vi "main.vi"() -> ()   [LabVIEW 2016]
uses:
  Typedefs/FGV_params.ctl
  Typedefs/FGV2_params.ctl
  Typedefs/State.ctl
  Typedefs/Acqstate.ctl
  <vilib>/Analysis/3filter.llb/Filter Passband Type.ctl
  <vilib>/DAQmx/read.llb/DAQmx Read (Analog 1D Wfm NChan NSamp).vi
  <vilib>/DAQmx/create/channels.llb/DAQmx Create Channel (AI-Voltage-Basic).vi
  <vilib>/DAQmx/configure/timing.llb/DAQmx Timing (Sample Clock).vi
  <vilib>/DAQmx/miscellaneous.llb/DAQmx Fill In Error Info.vi
  <vilib>/Analysis/3filter.llb/Butterworth Filter (DBL).vi
  <vilib>/Analysis/NI_AALBase.lvlib
panel:
  out "XZ":dbl(knob) scale=-90.0..90.0
  out "YZ":dbl(knob) scale=-90.0..90.0
  in  "Load?":bool
  in  "Save?":bool
  in  "Path?":path
  out "Acceleragement":waveform(dbl)[](graph)
  out "MAXY":dbl[](array[numeric])
  out "MINY":dbl[](array[numeric])
  in  "Axis?":string(combo)
  in  "Calibrate?":bool
  out "Voltagement":waveform(dbl)[](graph)
  in  "rate":dbl=1000.0 format="%0.2f"
  in  "samples per channel":i32=1000
  in  "stop":bool
  in  "Play?":bool
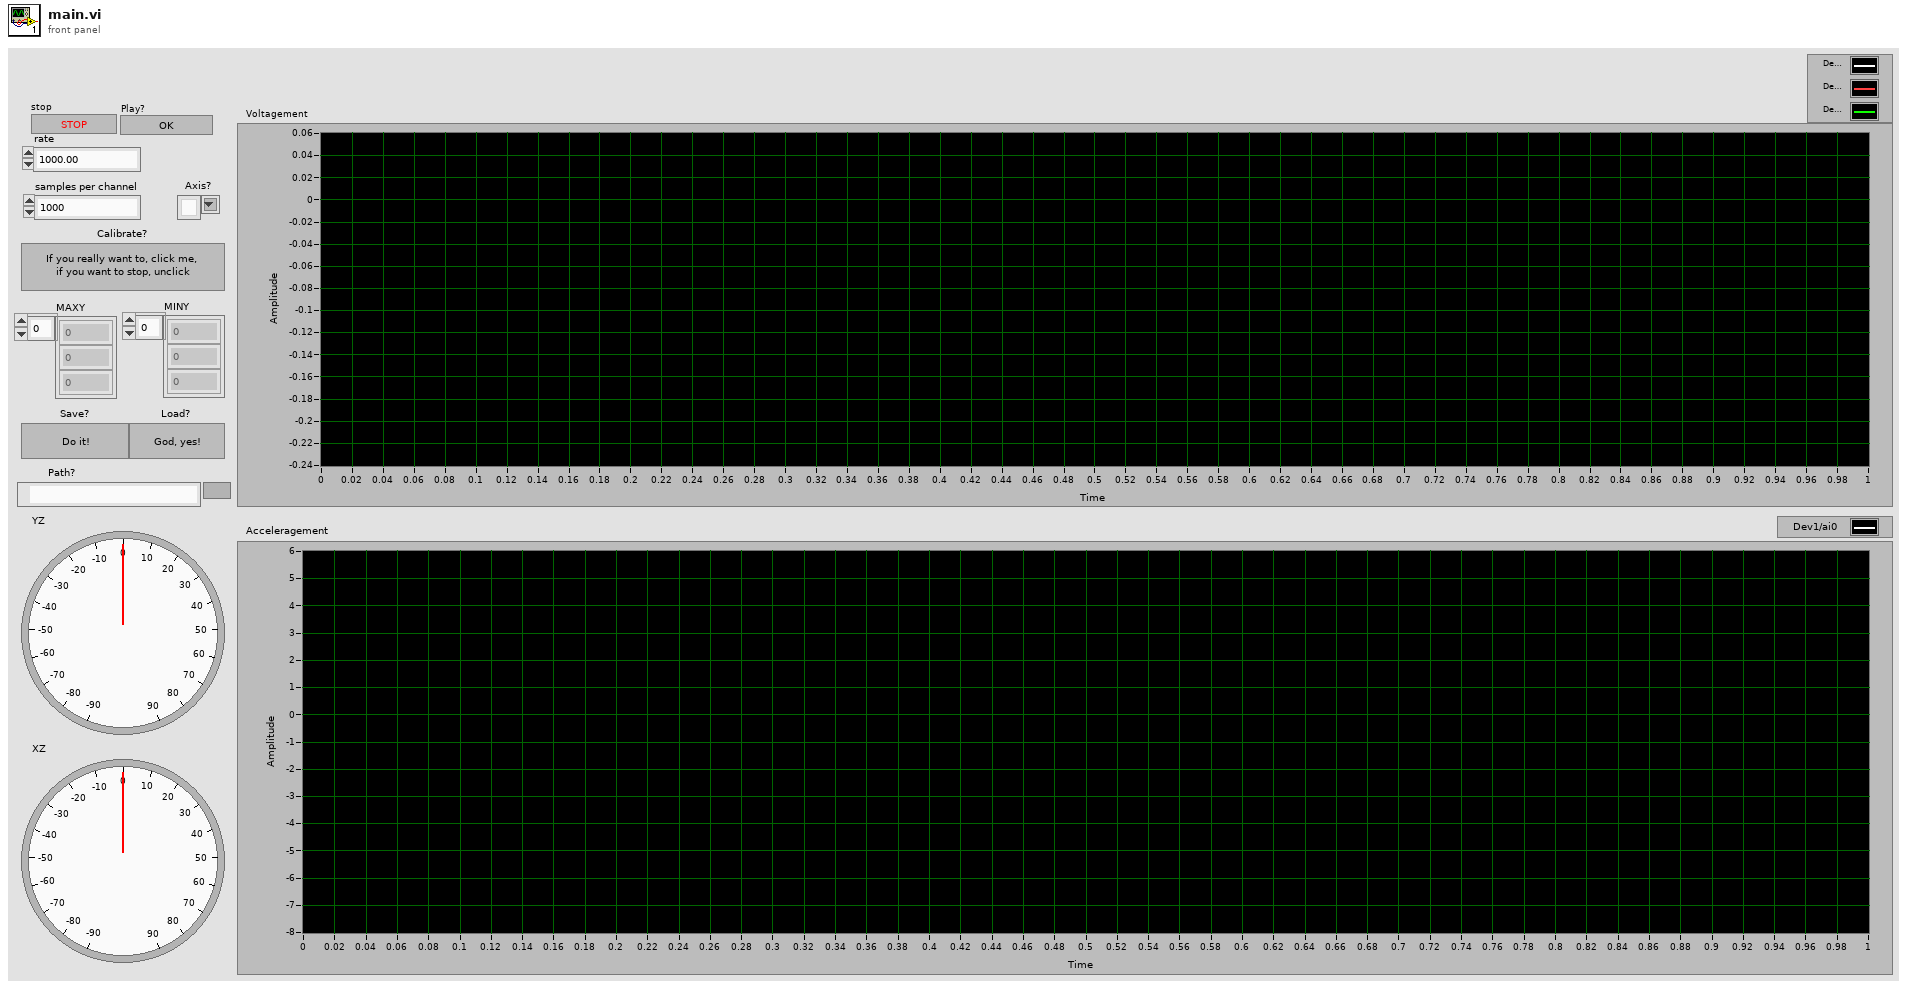
[diagram p1: front panel]
types:
  T1 = typedef "FGV2_params.ctl" = cluster{"Axis?":string, "Calibrate?":bool}
  T2 = typedef "FGV_params.ctl" = cluster{"Play":bool, "rate":dbl, "samples per channel":i32}
  T3 = typedef "Acqstate.ctl" = enum16{"Load", "Save", "Init", "Measurment", "Calibration"}
  T4 = typedef "State.ctl" = enum16{"Idel", "Init", "Acc", "End", ""}
  T5 = enum16{"open", "replace", "create", "open or create", "replace or create", "replace or create with confirmation"}
  T6 = typedef "NI_AALBase.lvlib/Filter Passband Type.ctl" = enum32{"Lowpass", "Highpass", "Bandpass", "Bandstop"}
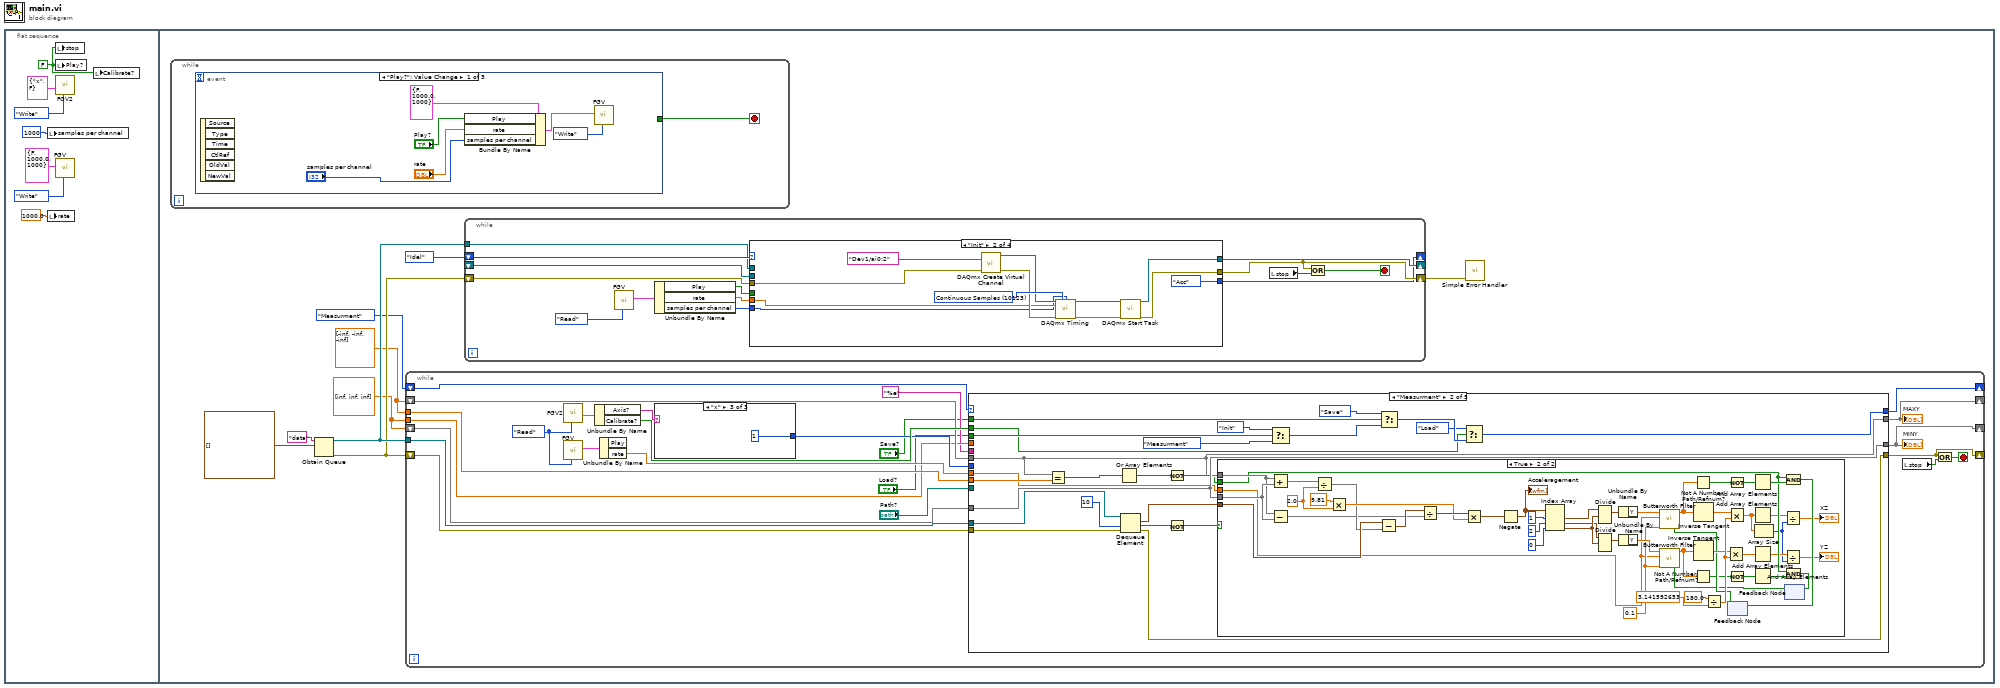
[diagram p0: block diagram]
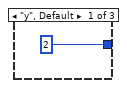
[diagram p2: hidden frame]
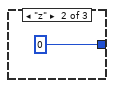
[diagram p3: hidden frame]
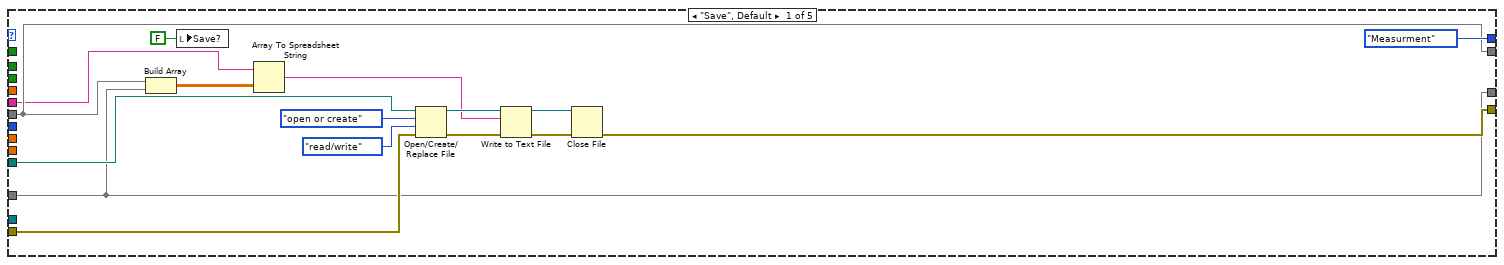
[diagram p4: hidden frame]
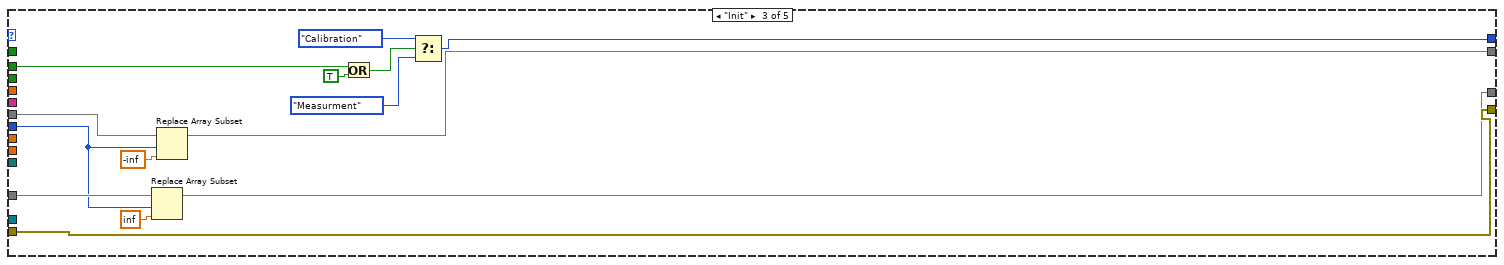
[diagram p6: hidden frame]
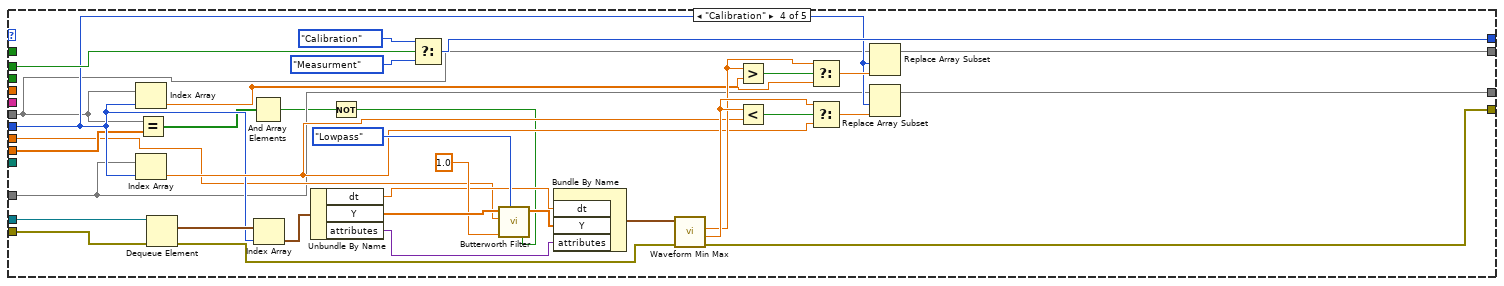
[diagram p7: hidden frame]
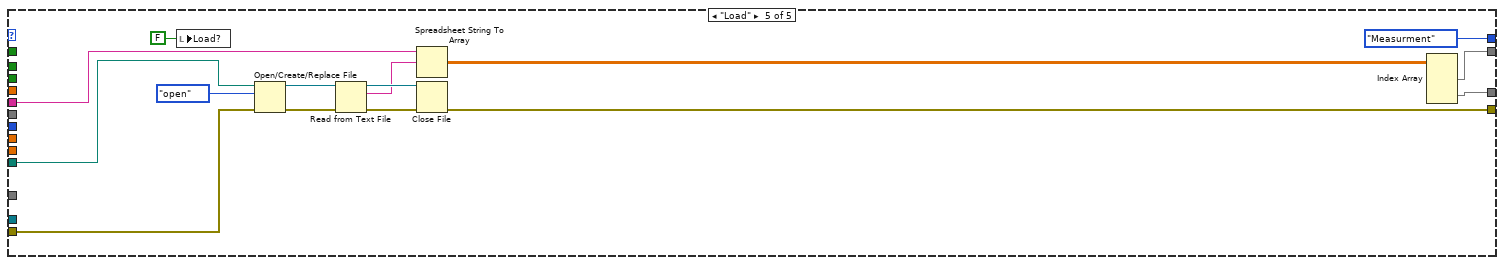
[diagram p8: hidden frame]
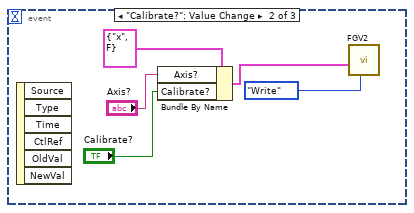
[diagram p9: hidden frame]
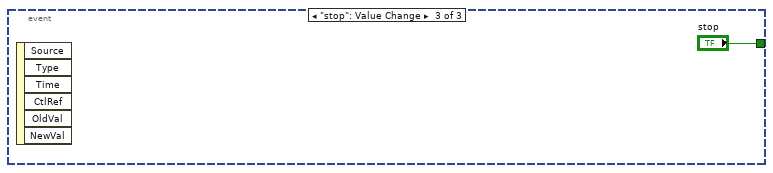
[diagram p10: hidden frame]
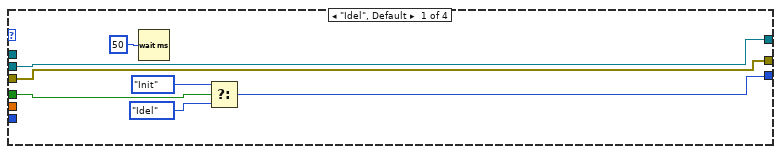
[diagram p11: hidden frame]
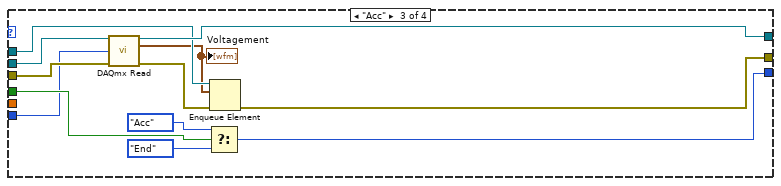
[diagram p12: hidden frame]
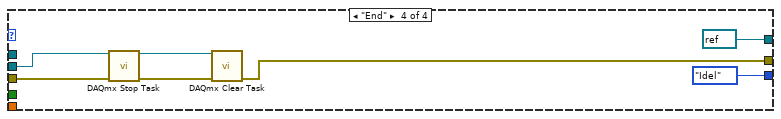
[diagram p13: hidden frame]
diagram:
  n1 = flat-sequence {
    frame #0 {
      w5 = FALSE
      n2 = local write "samples per channel"(1000 ("samples per channel")) -> ()
      n3 = local write "rate"(1000.0 ("rate")) -> ()
      n4 = local write "stop"(w5) -> ()
      n5 = local write "Play?"(w5) -> ()
      n6 = call "FGV2.vi"("Enum"=enum16{"Write", "Read"}."Write", "IN"=T1 {"Axis?"="x", "Calibrate?"=FALSE}) -> ()  [unwired: 8 in, 1 out]
      n7 = call "FGV.vi"("Enum"=enum16{"Write", "Read"}."Write", "IN"=T2 {"Play"=FALSE, "rate"=1000.0, "samples per channel"=1000}) -> ()  [unwired: 8 in, 1 out]
      n8 = local write "Calibrate?"(w5) -> ()
    }
    frame #1 {
      w9 = dbl[] [inf, inf, inf]
      w10 = dbl[] [-inf, -inf, -inf]
      n9 = while {
        stop <- w198 stop-if-true
        n10 = event shown="[0] \"Play?\": Value Change" {
          selector: _ -> [_ _ _]
          dyn-events: _ -> [_ _ _]
          timeout: _ -> [_ _ _]
          tunnel: [_ _ "stop"] -> w198
          event "Play?": Value Change {
            n11 = event-data() -> ()  [unwired: 1 in, 6 out]
            n12 = Bundle By Name(cluster=T2 {"Play"=FALSE, "rate"=1000.0, "samples per channel"=1000} ("IN"), "Play"="Play?", "rate"="rate", "samples per channel"="samples per channel") -> (w202:T2)
            n13 = call "FGV.vi"("Enum"=enum16{"Write", "Read"}."Write", "IN"=w202) -> ()  [unwired: 8 in, 1 out]
          }
          event "Calibrate?": Value Change {
            n14 = event-data() -> ()  [unwired: 1 in, 6 out]
            n15 = Bundle By Name(cluster=T1 {"Axis?"="x", "Calibrate?"=FALSE} ("IN"), "Axis?"="Axis?", "Calibrate?"="Calibrate?") -> (w207:T1)
            n16 = call "FGV2.vi"("Enum"=enum16{"Write", "Read"}."Write", "IN"=w207) -> ()  [unwired: 8 in, 1 out]
          }
          event "stop": Value Change {
            n17 = event-data() -> ()  [unwired: 1 in, 6 out]
          }
        }
      }
      n18 = Obtain Queue(name (unnamed)="data", element data type=waveform(dbl)[] [] ("data")) -> (queue out=w14:refnum<queue>, error out=w13:errorcluster)  [unwired: 3 in, 1 out]
      n19 = while {
        tunnel: w14 -> [w39]
        shift-right: [w36] -> _
        shift-left: w13 -> [w38]
        shift-right: [w24] -> _
        shift-left: w10 -> [w29]
        shift-right: [w25] -> _
        shift-left: w9 -> [w30]
        tunnel: w10 -> [w26]
        tunnel: w9 -> [w23]
        shift-right: [w20] -> _
        shift-left: Acqstate."Measurment" -> [w22]
        stop <- w37 stop-if-true
        w33 = enum16{"Write", "Read"}."Read" ("Enum")
        n20 = call "FGV2.vi"("Enum"=w33) -> ("OUT"=w32:T1)  [unwired: 9 in]
        n21 = call "FGV.vi"("Enum"=w33) -> ("OUT"=w40:T2)  [unwired: 9 in]
        n22 = Unbundle By Name(w32) -> ("Axis?"=w28:string, "Calibrate?"=w31:bool)
        n23 = Unbundle By Name(w40) -> ("rate"=w34:dbl)  [unwired: 1 out]
        n24 = case shown="\"x\"" w28 {
          tunnel: [2 ("Y max") 0 ("Y max") 1 ("Y max")] -> w27
          frame "y", Default {
          }
          frame "z" {
          }
          frame "x" {
          }
        }
        n25 = case shown="\"Measurment\"" w22 {
          tunnel: [Acqstate."Measurment" w62 w147 w182 Acqstate."Measurment"] -> w20
          tunnel: w39 -> [_ w80 _ w181 _]
          tunnel: w38 -> [w56 w79 w146 w180 w192]
          tunnel: [w49 w77 w146 w156 w193] -> w36
          tunnel: w34 -> [_ w72 _ w154 _]
          tunnel: w31 -> [_ w81 w138 w175 _]
          tunnel: [w47 w78 w142 w161 w187] -> w25
          tunnel: [w48 w74 w145 w162 w188] -> w24
          tunnel: w30 -> [w47 w78 w143 w152 _]
          tunnel: w29 -> [w48 w74 w144 w153 _]
          tunnel: w27 -> [_ _ w141 w159 _]
          tunnel: w26 -> [_ w75 _ w158 _]
          tunnel: w23 -> [_ _ _ _ _]
          tunnel: "Save?" -> [_ w64 _ _ _]
          tunnel: "Load?" -> [_ w60 _ _ _]
          tunnel: "Path?" -> [w51 _ _ _ w191]
          tunnel: "%e" ("format string") -> [w46 _ _ _ w185]
          frame "Save", Default {
            n26 = Build Array(w48, w47) -> (w53:dbl[][])
            n27 = local write "Save?"(FALSE) -> ()
            n28 = Array To Spreadsheet String(array=w53, 3:w46) -> (spreadsheet string=w52:string)  [unwired: 1 in]
            n29 = Open/Create/Replace File(file path (use dialog)=w51, error in=w56, operation (0:open)=T5."open or create", access (0:read/write)=enum16{"read/write", "read-only", "write-only"}."read/write") -> (refnum out=w58:refnum<file>, error out=w57:errorcluster)  [unwired: 2 in, 1 out]
            n30 = Write to Text File(file (use dialog)=w58, text=w52, error in=w57) -> (refnum out=w54:refnum<file>, error out=w55:errorcluster)  [unwired: 1 in, 1 out]
            n31 = Close File(refnum=w54, error in=w55) -> (error out=w49:errorcluster)  [unwired: 1 out]
          }
          frame "Measurment" {
            n32 = Equal?(x=w74, y=w75) -> (x = y?=w73:bool[])
            n33 = Or Array Elements(Boolean array=w73) -> (logical OR=w71:bool)
            n34 = Dequeue Element(queue=w80, timeout in ms (-1)=10, error in (no error)=w79) -> (element=w76:waveform(dbl)[], timed out?=w67:bool, error out=w77:errorcluster)  [unwired: 1 out]
            n35 = Not(x=w71) -> (.not. x?=w70:bool)
            n36 = Not(x=w67) -> (.not. x?=w68:bool)
            n37 = case shown="True" w68 {
              tunnel: w78 -> [_ w133]
              tunnel: w76 -> [_ w132]
              tunnel: w74 -> [_ w105]
              tunnel: w72 -> [_ w104]
              tunnel: w70 -> [_ w92]
              frame False {
              }
              frame True {
                w106 = 0.1 ("low cutoff freq: fl")
                w127 = 2.0 ("y")
                n38 = Add(x=w105, y=w133) -> (x+y=w126:dbl[])
                n39 = Subtract(x=w105, y=w133) -> (x-y=w124:dbl[])
                n40 = Divide(x=w126, y=w127) -> (x/y=w128:dbl[])
                n41 = Multiply(x=9.81, y=w127) -> (x*y=w129:dbl)
                n42 = Subtract(x=w132, y=w128) -> (x-y=w125:waveform(dbl)[])
                n43 = Divide(x=w125, y=w124) -> (x/y=w131:waveform(dbl)[])
                n44 = Multiply(x=w131, y=w129) -> (x*y=w123:waveform(dbl)[])
                n45 = Negate(x=w123) -> (-x=w122:waveform(dbl)[])
                "Acceleragement" <- w122
                n46 = Index Array(array=w122, index #1=1 ("index"), index #2=2 ("index"), index #3=0 ("index")) -> (element #1=w111:waveform(dbl), element #2=w109:waveform(dbl), element #3=w110:waveform(dbl))
                n47 = Divide(1:w110, 2:w111) -> (0:w114:waveform(dbl))  [unwired: 1 in, 1 out]
                n48 = Divide(1:w110, 2:w109) -> (0:w113:waveform(dbl))  [unwired: 1 in, 1 out]
                n49 = Unbundle By Name(w114) -> ("Y"=w108:dbl[])
                n50 = Unbundle By Name(w113) -> ("Y"=w107:dbl[])
                n51 = Divide(x=180.0, y=3.141592653) -> (x/y=w116:dbl)
                n52 = feedback #1() -> (w98:bool)  [unwired: 1 in]
                n53 = call-poly <vilib>:"Butterworth Filter.vi"("init/cont (init:F)"=w98, "low cutoff freq: fl"=w106, "sampling freq: fs"=w104, "X"=w108) -> ("Filtered X"=w103:dbl[])  [unwired: 4 in, 1 out]
                n54 = Not A Number/Path/Refnum?(number/path/refnum=w103) -> (NaN/Path/Refnum?=w102:bool[])
                n55 = Inverse Tangent(1:w103) -> (0:w115:dbl[])
                n56 = Not(x=w102) -> (.not. x?=w101:bool[])
                n57 = Multiply(x=w115, y=w116) -> (x*y=w89:dbl[])
                n58 = And Array Elements(Boolean array=w101) -> (logical AND=w100:bool)
                n59 = Add Array Elements(numeric array=w89) -> (sum=w88:dbl)
                n60 = Array Size(array=w89) -> (size(s)=w85:i32)
                n61 = Divide(x=w88, y=w85) -> (x/y=→"XZ":dbl)
                n62 = And(x=w92, y=w100) -> (x .and. y?=w99:bool)
                n63 = feedback-in #1(w99) -> ()
                n64 = feedback #2() -> (w91:bool)  [unwired: 1 in]
                n65 = call-poly <vilib>:"Butterworth Filter.vi"("init/cont (init:F)"=w91, "low cutoff freq: fl"=w106, "sampling freq: fs"=w104, "X"=w107) -> ("Filtered X"=w93:dbl[])  [unwired: 4 in, 1 out]
                n66 = Not A Number/Path/Refnum?(number/path/refnum=w93) -> (NaN/Path/Refnum?=w97:bool[])
                n67 = Inverse Tangent(1:w93) -> (0:w112:dbl[])
                n68 = Multiply(x=w112, y=w116) -> (x*y=w90:dbl[])
                n69 = Not(x=w97) -> (.not. x?=w96:bool[])
                n70 = Add Array Elements(numeric array=w90) -> (sum=w86:dbl)
                n71 = And Array Elements(Boolean array=w96) -> (logical AND=w95:bool)
                n72 = Divide(x=w86, y=w85) -> (x/y=→"YZ":dbl)
                n73 = And(x=w92, y=w95) -> (x .and. y?=w94:bool)
                n74 = feedback-in #2(w94) -> ()
              }
            }
            n75 = Select(t=Acqstate."Init", s=w81, f=Acqstate."Measurment") -> (s? t:f=w66:T3)
            n76 = Select(t=Acqstate."Save", s=w64, f=w66) -> (s? t:f=w63:T3)
            n77 = Select(t=Acqstate."Load", s=w60, f=w63) -> (s? t:f=w62:T3)
          }
          frame "Init" {
            n78 = Replace Array Subset(array=w143, new element=inf ("new element/subarray"), index=w141) -> (w142:dbl[])
            n79 = Replace Array Subset(array=w144, new element=-inf ("new element/subarray"), index=w141) -> (w145:dbl[])
            n80 = Or(x=w138, y=TRUE) -> (x .or. y?=w137:bool)
            n81 = Select(t=Acqstate."Calibration", s=w137, f=Acqstate."Measurment") -> (s? t:f=w147:T3)
          }
          frame "Calibration" {
            n82 = Index Array(array=w153, index=w159) -> (element=w164:dbl)
            n83 = Index Array(array=w152, index=w159) -> (element=w165:dbl)
            n84 = Equal?(x=w153, y=w158) -> (x = y?=w157:bool[])
            n85 = Dequeue Element(queue=w181, error in (no error)=w180) -> (element=w179:waveform(dbl)[], error out=w155:errorcluster)  [unwired: 1 in, 2 out]
            n86 = And Array Elements(Boolean array=w157) -> (logical AND=w150:bool)
            n87 = Index Array(array=w179, index=w159) -> (element=w174:waveform(dbl))
            n88 = Unbundle By Name(w174) -> ("dt"=w169:dbl, "Y"=w178:dbl[], "attributes"=w167:variant)
            n89 = Not(x=w150) -> (.not. x?=w151:bool)
            n90 = Select(t=Acqstate."Calibration", s=w175, f=Acqstate."Measurment") -> (s? t:f=w182:T3)
            n91 = call-poly <vilib>:"Butterworth Filter.vi"("init/cont (init:F)"=w151, "filter type"=Filter_Passband_Type."Lowpass", "low cutoff freq: fl"=1.0, "sampling freq: fs"=w154, "X"=w178) -> ("Filtered X"=w168:dbl[])  [unwired: 3 in, 1 out]
            n92 = Bundle By Name("dt"=w169, "Y"=w168, "attributes"=w167) -> (w166:waveform(dbl))  [unwired: 1 in]
            n93 = call <vilib>:"Waveform Min Max.vi"("error in (no error)"=w155, "waveform in"=w166) -> ("error out"=w156:errorcluster, "Y min"=w172:dbl, "Y max"=w170:dbl)  [unwired: 4 in, 3 out]
            n94 = Greater?(x=w170, y=w164) -> (0:w171:bool)
            n95 = Less?(x=w172, y=w165) -> (x < y?=w173:bool)
            n96 = Select(t=w170, s=w171, f=w164) -> (s? t:f=w163:dbl)
            n97 = Select(t=w172, s=w173, f=w165) -> (s? t:f=w160:dbl)
            n98 = Replace Array Subset(array=w153, new element=w163, index=w159) -> (w162:dbl[])
            n99 = Replace Array Subset(array=w152, new element=w160, index=w159) -> (w161:dbl[])
          }
          frame "Load" {
            n100 = local write "Load?"(FALSE) -> ()
            n101 = Open/Create/Replace File(file path (use dialog)=w191, error in=w192, operation (0:open)=T5."open") -> (refnum out=w197:refnum<file>, error out=w196:errorcluster)  [unwired: 3 in, 1 out]
            n102 = Read from Text File(file (use dialog)=w197, error in=w196) -> (refnum out=w194:refnum<file>, text=w190:string, error out=w195:errorcluster)  [unwired: 2 in, 1 out]
            n103 = Spreadsheet String To Array(format string=w185, spreadsheet string=w190) -> (array=w189:dbl[][])  [unwired: 2 in]
            n104 = Close File(refnum=w194, error in=w195) -> (error out=w193:errorcluster)  [unwired: 1 out]
            n105 = Index Array(array=w189) -> (element #1=w188:dbl[], element #2=w187:dbl[])  [unwired: 4 in]
          }
        }
        "MINY" <- w25
        "MAXY" <- w24
        n106 = local read "stop"() -> (w35:bool)
        n107 = Or(x=w36, y=w35) -> (x .or. y?=w37:bool)
      }
      n108 = while {
        shift-right: [w212] -> _
        shift-left: State."Idel" -> [w224]
        shift-right: [w221] -> w15
        shift-left: w13 -> [w220]
        shift-right: [w222] -> _
        shift-left: _ -> [w219]
        tunnel: w14 -> [w211]
        stop <- w223 stop-if-true
        n109 = call "FGV.vi"("Enum"=enum16{"Write", "Read"}."Read") -> ("OUT"=w216:T2)  [unwired: 9 in]
        n110 = Unbundle By Name(w216) -> ("Play"=w215:bool, "rate"=w214:dbl, "samples per channel"=w213:i32)
        n111 = case shown="\"Init\"" w224 {
          tunnel: [w228 State."Acc" w250 State."Idel"] -> w212
          tunnel: [w226 w240 w253 refnum<k21> refnum ("task out")] -> w222
          tunnel: [w227 w239 w245 w260] -> w221
          tunnel: w220 -> [w227 w236 w254 w257]
          tunnel: w219 -> [w226 _ w255 w258]
          tunnel: w215 -> [w225 _ w249 _]
          tunnel: w214 -> [_ w234 _ _]
          tunnel: w213 -> [_ w233 w248 _]
          tunnel: w211 -> [_ _ w247 _]
          frame "Idel", Default {
            n112 = Wait (ms)(milliseconds to wait=u32 50) -> ()  [unwired: 1 out]
            n113 = Select(t=State."Init", s=w225, f=State."Idel") -> (s? t:f=w228:T4)
          }
          frame "Init" {
            w243 = 10123 items=["Finite Samples"=10178, "Continuous Samples"=10123, "Hardware Timed Single Point"=12522] ("sample mode")
            n114 = call-poly <vilib>:"DAQmx Create Virtual Channel.vi"("physical channels"=tag "Dev1/ai0:2", "error in"=w236) -> ("task out"=w238:refnum<k21>, "error out"=w237:errorcluster)  [unwired: 12 in]
            n115 = call-poly <vilib>:"DAQmx Timing.vi"("task/channels in"=w238, "sample mode"=w243, "samples per channel"=w233, "rate"=w234, "error in"=w237) -> ("task out"=w242:refnum<k21>, "error out"=w241:errorcluster)  [unwired: 9 in]
            n116 = call <vilib>:"DAQmx Start Task.vi"("task/channels in"=w242, "error in"=w241) -> ("task out"=w240:refnum<k21>, "error out"=w239:errorcluster)  [unwired: 12 in]
          }
          frame "Acc" {
            n117 = call-poly <vilib>:"DAQmx Read.vi"("task/channels in"=w255, "number of samples per channel"=w248, "error in"=w254) -> ("task out"=w253:refnum<k21>, "data"=w244:waveform(dbl)[], "error out"=w246:errorcluster)  [unwired: 10 in]
            "Voltagement" <- w244
            n118 = Select(t=State."Acc", s=w249, f=State."End") -> (s? t:f=w250:T4)
            n119 = Enqueue Element(queue=w247, element=w244, error in (no error)=w246) -> (error out=w245:errorcluster)  [unwired: 1 in, 2 out]
          }
          frame "End" {
            n120 = call <vilib>:"DAQmx Stop Task.vi"("task/channels in"=w258, "error in"=w257) -> ("task out"=w262:refnum<k21>, "error out"=w261:errorcluster)  [unwired: 12 in]
            n121 = call <vilib>:"DAQmx Clear Task.vi"("task in"=w262, "error in"=w261) -> ("error out"=w260:errorcluster)  [unwired: 13 in]
          }
        }
        n122 = local read "stop"() -> (w218:bool)
        n123 = Or(x=w221, y=w218) -> (x .or. y?=w223:bool)
      }
      n124 = call <vilib>:"Simple Error Handler.vi"("error in (no error)"=w15) -> ()  [unwired: 4 in, 5 out]
    }
  }
